vi "MarbleDispenserMk6.vi"() -> ()   [LabVIEW 2016]
uses:
  <vilib>/NXT/Block Support/NXT_InputPort.ctl
  <vilib>/NXT/Block Support/NXT_OutputPort.ctl
  <vilib>/NXT/Dual Mode Library/Sensors/Touch_Released.vi
  <vilib>/NXT/NXTIO Xnodes/NXTIONodeSubVIs/NXTStopMotors.vi
  <vilib>/NXT/NXTIO Xnodes/NXTIONodeSubVIs/NXTMotorRunDistance.vi
  <vilib>/NXT/Dual Mode Library/Waits/Wait_Num.vi
  <vilib>/NXT/Dual Mode Library/Sensors/Touch_Pressed.vi
  <vilib>/NXT/Dual Mode Library/Sensors/EV3_Color_Color.vi
  <vilib>/NXT/Subs/LVHSConnector.ctl
  <vilib>/NXT/NXTIO Xnodes/AddressXNode/NXTIOAddress.xnode
  <vilib>/NXT/NXTIO Xnodes/NXTIOXNode/NXTIO.xnode
  <vilib>/NXT/LegoClasses/BrickReference/BrickReference.lvclass
panel:
  out "Distance":dbl
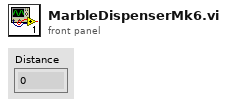
[diagram p1: front panel]
types:
  T1 = typedef "NXT_InputPort.ctl" = u32
  T2 = typedef "NXT_OutputPort.ctl" = u8
  T3 = typedef "LVHSConnector.ctl" = refnum<class "BrickReference.lvclass">
  T4 = typedef "ColorSensorColors.ctl" = enum16{"No Color", "Black", "Blue", "Green", "Yellow", "Red", "White", "Brown"}
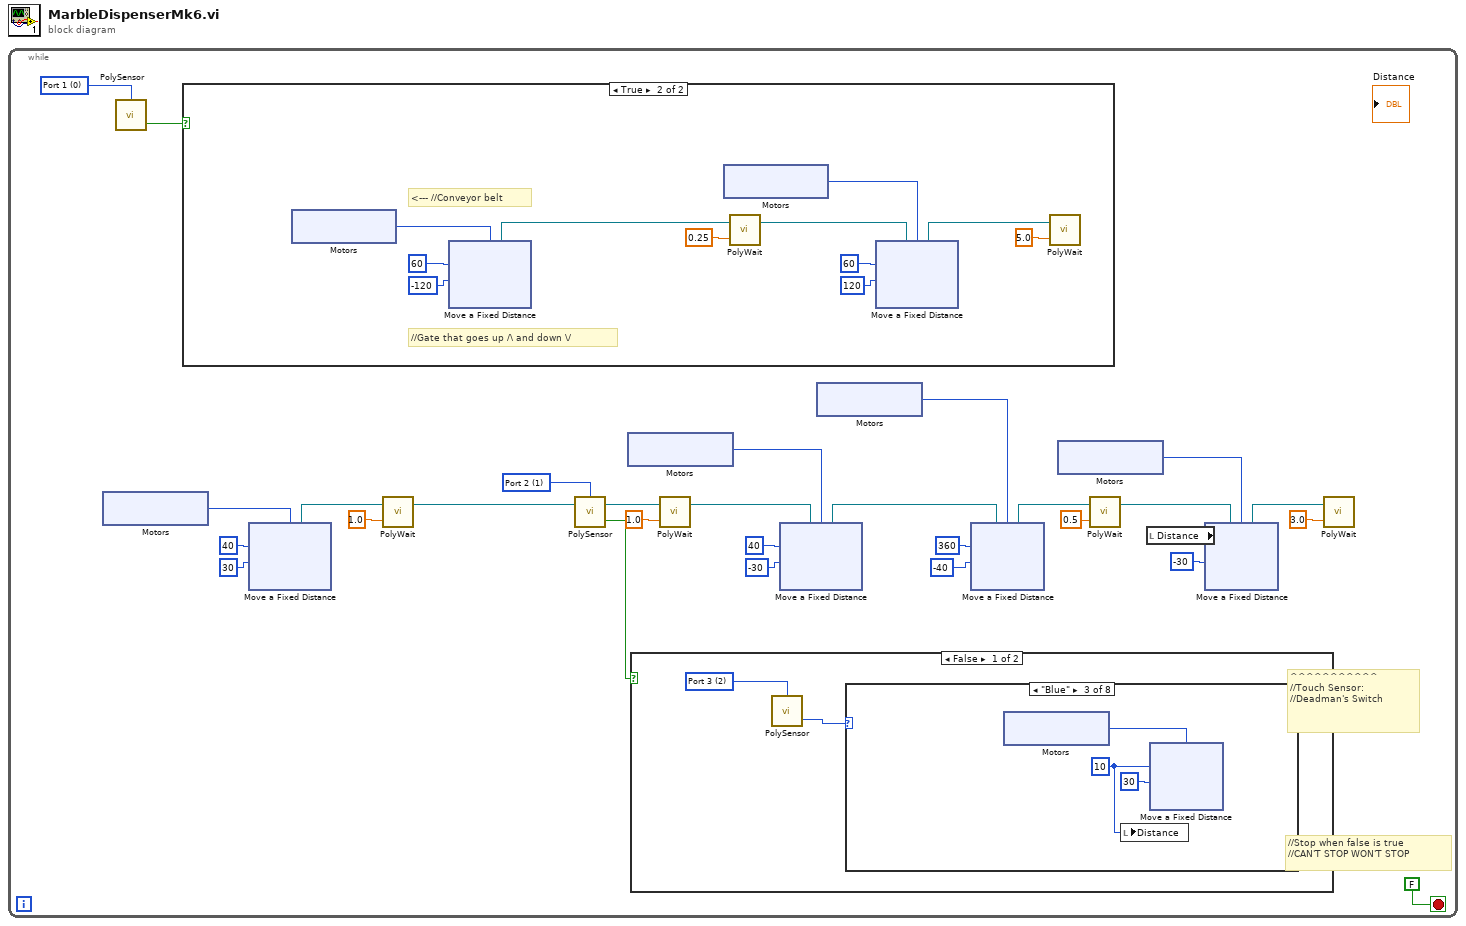
[diagram p0: block diagram]
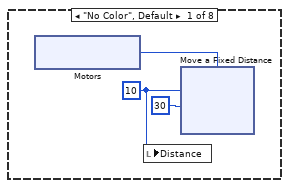
[diagram p2: hidden frame]
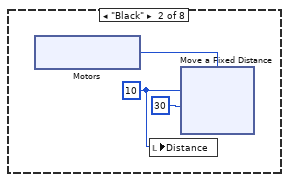
[diagram p3: hidden frame]
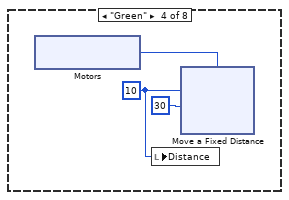
[diagram p4: hidden frame]
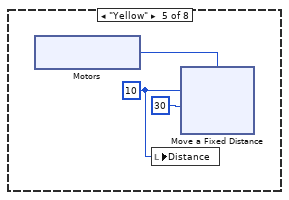
[diagram p5: hidden frame]
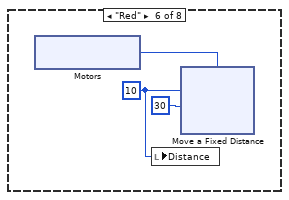
[diagram p6: hidden frame]
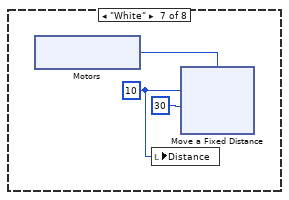
[diagram p7: hidden frame]
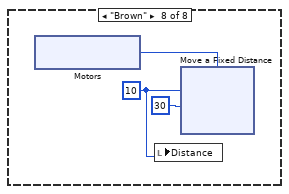
[diagram p8: hidden frame]
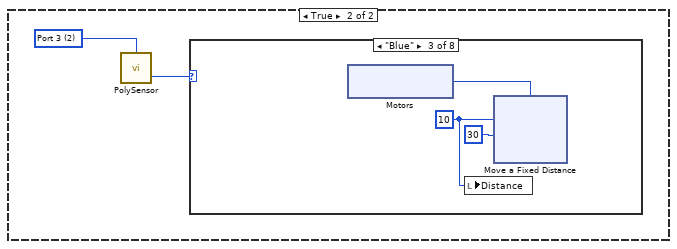
[diagram p9: hidden frame]
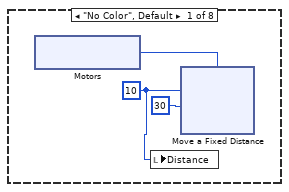
[diagram p10: hidden frame]
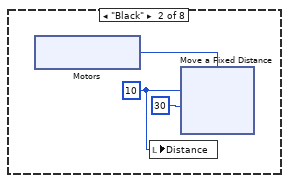
[diagram p11: hidden frame]
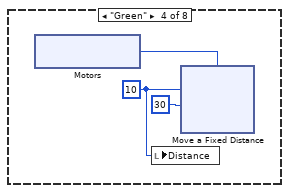
[diagram p12: hidden frame]
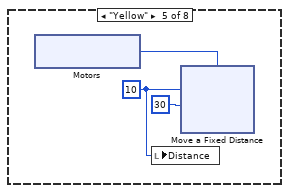
[diagram p13: hidden frame]
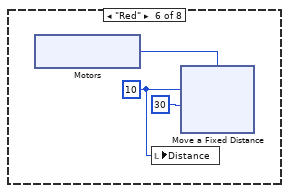
[diagram p14: hidden frame]
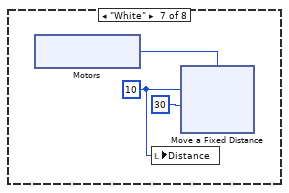
[diagram p15: hidden frame]
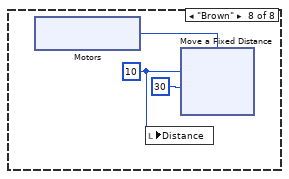
[diagram p16: hidden frame]
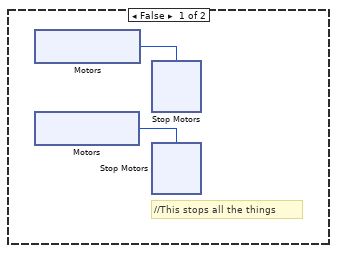
[diagram p17: hidden frame]
diagram:
  n1 = while {
    stop <- FALSE stop-if-true
    w16 = T1 1 items=["Port 1", "Port 2", "Port 3", "Port 4"] ("Port (Port 1)")
    w29 = T1 0 items=["Port 1", "Port 2", "Port 3", "Port 4"] ("Port (Port 1)")
    # "//Stop when false is true\n//CAN'T STOP WON'T STOP"
    # "^^^^^^^^^^^\n//Touch Sensor:\n//Deadman's Switch"
    n2 = xnode "Motors"() -> ("Motor"=w22:T2)
    n3 = call-poly <vilib>:"PolySensor.vi"("Port (Port 1)"=w29) -> ("Yes / No"=w27:bool)  [unwired: 2 in, 1 out]
    n4 = case shown="True" w27 {
      frame False {
        # "//This stops all the things"
        n5 = xnode "Motors"() -> ("Motor"=w303:T2)
        n6 = xnode "Motors"() -> ("Motor"=w302:T2)
        n7 = xnode "Stop Motors"("Motors"=w303) -> ()  [unwired: 1 in, 1 out]
        n8 = xnode "Stop Motors"("Motors"=w302) -> ()  [unwired: 1 in, 1 out]
      }
      frame True {
        # "//Gate that goes up /\\ and down \\/"
        # "<--- //Conveyor belt"
        n9 = xnode "Motors"() -> ("Motor"=w322:T2)
        n10 = xnode "Move a Fixed Distance"("Speed 1"=-120, "Distance 1"=60, "Motors"=w322) -> ("NXT/EV3"=w325:T3)  [unwired: 1 in]
        n11 = xnode "Motors"() -> ("Motor"=w316:T2)
        n12 = call-poly <vilib>:"PolyWait.vi"("Time (1 sec)"=0.25, "NXT/EV3"=w325) -> ("NXT/EV3"=w317:T3)  [unwired: 2 in]
        n13 = xnode "Move a Fixed Distance"("Speed 1"=120, "Distance 1"=60, "Motors"=w316, "NXT/EV3"=w317) -> ("NXT/EV3"=w320:T3)
        n14 = call-poly <vilib>:"PolyWait.vi"("Time (1 sec)"=5.0, "NXT/EV3"=w320) -> ()  [unwired: 2 in, 1 out]
      }
    }
    n15 = xnode "Move a Fixed Distance"("Speed 1"=30, "Distance 1"=40, "Motors"=w22) -> ("NXT/EV3"=w25:T3)  [unwired: 1 in]
    n16 = call-poly <vilib>:"PolyWait.vi"("Time (1 sec)"=1.0, "NXT/EV3"=w25) -> ("NXT/EV3"=w17:T3)  [unwired: 2 in]
    n17 = call-poly <vilib>:"PolySensor.vi"("NXT/EV3"=w17, "Port (Port 1)"=w16) -> ("Yes / No"=w15:bool, "NXT/EV3"=w14:T3)  [unwired: 1 in]
    n18 = xnode "Motors"() -> ("Motor"=w18:T2)
    n19 = case shown="False" w15 {
      frame False {
        w52 = T1 2 items=["Port 1", "Port 2", "Port 3", "Port 4"] ("Port (Port 1)")
        n20 = call-poly <vilib>:"PolySensor.vi"("Port (Port 1)"=w52) -> ("Detected Color"=w53:T4)  [unwired: 2 in, 1 out]
        n21 = case shown="\"Blue\"" w53 {
          frame "No Color", Default {
            w54 = 10 ("Distance 1")
            n22 = xnode "Motors"() -> ("Motor"=w55:T2)
            n23 = local write "Distance"(w54) -> ()
            n24 = xnode "Move a Fixed Distance"("Speed 1"=i8 30, "Distance 1"=w54, "Motors"=w55) -> ()  [unwired: 1 in, 1 out]
          }
          frame "Black" {
            w68 = 10 ("Distance 1")
            n25 = xnode "Motors"() -> ("Motor"=w69:T2)
            n26 = local write "Distance"(w68) -> ()
            n27 = xnode "Move a Fixed Distance"("Speed 1"=i8 30, "Distance 1"=w68, "Motors"=w69) -> ()  [unwired: 1 in, 1 out]
          }
          frame "Blue" {
            w82 = 10 ("Distance 1")
            n28 = xnode "Motors"() -> ("Motor"=w84:T2)
            n29 = local write "Distance"(w82) -> ()
            n30 = xnode "Move a Fixed Distance"("Speed 1"=i8 30, "Distance 1"=w82, "Motors"=w84) -> ()  [unwired: 1 in, 1 out]
          }
          frame "Green" {
            w96 = 10 ("Distance 1")
            n31 = xnode "Motors"() -> ("Motor"=w98:T2)
            n32 = local write "Distance"(w96) -> ()
            n33 = xnode "Move a Fixed Distance"("Speed 1"=i8 30, "Distance 1"=w96, "Motors"=w98) -> ()  [unwired: 1 in, 1 out]
          }
          frame "Yellow" {
            w110 = 10 ("Distance 1")
            n34 = xnode "Motors"() -> ("Motor"=w111:T2)
            n35 = local write "Distance"(w110) -> ()
            n36 = xnode "Move a Fixed Distance"("Speed 1"=i8 30, "Distance 1"=w110, "Motors"=w111) -> ()  [unwired: 1 in, 1 out]
          }
          frame "Red" {
            w124 = 10 ("Distance 1")
            n37 = xnode "Motors"() -> ("Motor"=w126:T2)
            n38 = local write "Distance"(w124) -> ()
            n39 = xnode "Move a Fixed Distance"("Speed 1"=i8 30, "Distance 1"=w124, "Motors"=w126) -> ()  [unwired: 1 in, 1 out]
          }
          frame "White" {
            w138 = 10 ("Distance 1")
            n40 = xnode "Motors"() -> ("Motor"=w140:T2)
            n41 = local write "Distance"(w138) -> ()
            n42 = xnode "Move a Fixed Distance"("Speed 1"=i8 30, "Distance 1"=w138, "Motors"=w140) -> ()  [unwired: 1 in, 1 out]
          }
          frame "Brown" {
            w152 = 10 ("Distance 1")
            n43 = xnode "Motors"() -> ("Motor"=w153:T2)
            n44 = local write "Distance"(w152) -> ()
            n45 = xnode "Move a Fixed Distance"("Speed 1"=i8 30, "Distance 1"=w152, "Motors"=w153) -> ()  [unwired: 1 in, 1 out]
          }
        }
      }
      frame True {
        w166 = T1 2 items=["Port 1", "Port 2", "Port 3", "Port 4"] ("Port (Port 1)")
        n46 = call-poly <vilib>:"PolySensor.vi"("Port (Port 1)"=w166) -> ("Detected Color"=w167:T4)  [unwired: 2 in, 1 out]
        n47 = case shown="\"Blue\"" w167 {
          frame "No Color", Default {
            w168 = 10 ("Distance 1")
            n48 = xnode "Motors"() -> ("Motor"=w169:T2)
            n49 = local write "Distance"(w168) -> ()
            n50 = xnode "Move a Fixed Distance"("Speed 1"=i8 30, "Distance 1"=w168, "Motors"=w169) -> ()  [unwired: 1 in, 1 out]
          }
          frame "Black" {
            w182 = 10 ("Distance 1")
            n51 = xnode "Motors"() -> ("Motor"=w183:T2)
            n52 = local write "Distance"(w182) -> ()
            n53 = xnode "Move a Fixed Distance"("Speed 1"=i8 30, "Distance 1"=w182, "Motors"=w183) -> ()  [unwired: 1 in, 1 out]
          }
          frame "Blue" {
            w196 = 10 ("Distance 1")
            n54 = xnode "Motors"() -> ("Motor"=w198:T2)
            n55 = local write "Distance"(w196) -> ()
            n56 = xnode "Move a Fixed Distance"("Speed 1"=i8 30, "Distance 1"=w196, "Motors"=w198) -> ()  [unwired: 1 in, 1 out]
          }
          frame "Green" {
            w210 = 10 ("Distance 1")
            n57 = xnode "Motors"() -> ("Motor"=w212:T2)
            n58 = local write "Distance"(w210) -> ()
            n59 = xnode "Move a Fixed Distance"("Speed 1"=i8 30, "Distance 1"=w210, "Motors"=w212) -> ()  [unwired: 1 in, 1 out]
          }
          frame "Yellow" {
            w224 = 10 ("Distance 1")
            n60 = xnode "Motors"() -> ("Motor"=w225:T2)
            n61 = local write "Distance"(w224) -> ()
            n62 = xnode "Move a Fixed Distance"("Speed 1"=i8 30, "Distance 1"=w224, "Motors"=w225) -> ()  [unwired: 1 in, 1 out]
          }
          frame "Red" {
            w238 = 10 ("Distance 1")
            n63 = xnode "Motors"() -> ("Motor"=w240:T2)
            n64 = local write "Distance"(w238) -> ()
            n65 = xnode "Move a Fixed Distance"("Speed 1"=i8 30, "Distance 1"=w238, "Motors"=w240) -> ()  [unwired: 1 in, 1 out]
          }
          frame "White" {
            w252 = 10 ("Distance 1")
            n66 = xnode "Motors"() -> ("Motor"=w254:T2)
            n67 = local write "Distance"(w252) -> ()
            n68 = xnode "Move a Fixed Distance"("Speed 1"=i8 30, "Distance 1"=w252, "Motors"=w254) -> ()  [unwired: 1 in, 1 out]
          }
          frame "Brown" {
            w266 = 10 ("Distance 1")
            n69 = xnode "Motors"() -> ("Motor"=w268:T2)
            n70 = local write "Distance"(w266) -> ()
            n71 = xnode "Move a Fixed Distance"("Speed 1"=i8 30, "Distance 1"=w266, "Motors"=w268) -> ()  [unwired: 1 in, 1 out]
          }
        }
      }
    }
    n72 = call-poly <vilib>:"PolyWait.vi"("Time (1 sec)"=sgl 1.0, "NXT/EV3"=w14) -> ("NXT/EV3"=w13:T3)  [unwired: 2 in]
    n73 = xnode "Move a Fixed Distance"("Speed 1"=-30, "Distance 1"=40, "Motors"=w18, "NXT/EV3"=w13) -> ("NXT/EV3"=w11:T3)
    n74 = xnode "Motors"() -> ("Motor"=w9:T2)
    n75 = xnode "Move a Fixed Distance"("Speed 1"=i8 -40, "Distance 1"=360, "Motors"=w9, "NXT/EV3"=w11) -> ("NXT/EV3"=w10:T3)
    n76 = xnode "Motors"() -> ("Motor"=w4:T2)
    n77 = call-poly <vilib>:"PolyWait.vi"("Time (1 sec)"=0.5, "NXT/EV3"=w10) -> ("NXT/EV3"=w5:T3)  [unwired: 2 in]
    n78 = local read "Distance"() -> (w1:dbl)
    n79 = xnode "Move a Fixed Distance"("Speed 1"=i8 -30, "Distance 1"=w1, "Motors"=w4, "NXT/EV3"=w5) -> ("NXT/EV3"=w3:T3)
    n80 = call-poly <vilib>:"PolyWait.vi"("Time (1 sec)"=3.0, "NXT/EV3"=w3) -> ()  [unwired: 2 in, 1 out]
  }
